vi "String Conversion.vi"(8 "추가할 문자열":string, 10 "문자열 입력":string) -> (2 "변경된 문자열 출력":string)   [LabVIEW 2020]
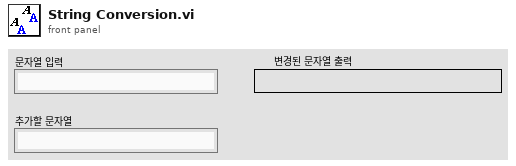
[diagram p1: front panel]
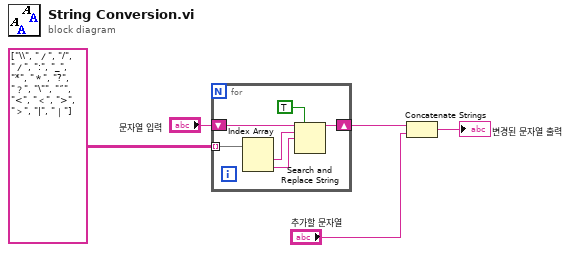
[diagram p0: block diagram]
diagram:
  n1 = for {
    tunnel: string[][] [["\\", "／"], ["/", "／"], [":", "_"], ["*", "＊"], ["?", "？"], ["\"", "˝"], ["<", "＜"], [">", "＞"], ["|", "｜"]] ("전치된 배열") -> [w9] mode=indexing
    shift-right: [w6] -> w3
    shift-left: "문자열 입력" -> [w11]
    n2 = Index Array(array=w9) -> (element #1=w8:string, element #2=w7:string)  [unwired: 2 in]
    n3 = Search and Replace String(replace all?=TRUE ("모두 대체? (거짓)"), input string=w11, search string=w8, replace string=w7) -> (result string=w6:string)  [unwired: 4 in, 3 out]
  }
  n4 = Concatenate Strings(w3, "추가할 문자열") -> (→"변경된 문자열 출력":string)
